vi "Create Dataset 2D Double.vi"(7 "Chunk size":i32, 8 "error in (no error)":errorcluster, 9 "Datatype":dbl[][](array[numeric]), 10 "Dataset name":string, 11 "Location id in":i32) -> (0 "error out":errorcluster, 3 "Dataset id":i32)   [LabVIEW 2014]
uses:
  Release/HDF5Tools.dll
  HDF5Tools.lvlib
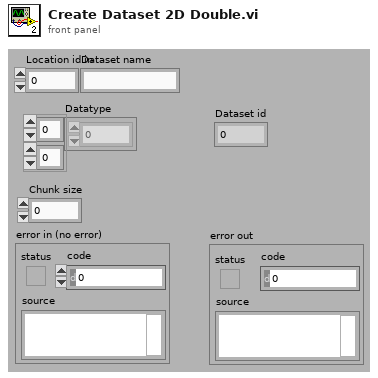
[diagram p1: front panel]
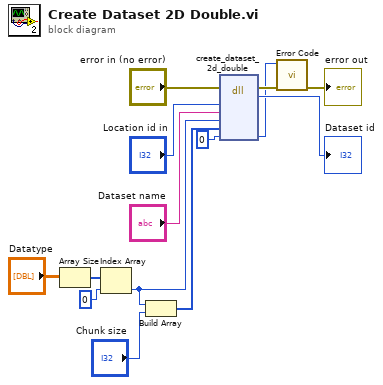
[diagram p0: block diagram]
diagram:
  n1 = Array Size(array="Datatype") -> (size(s)=w10:i32[])
  n2 = Index Array(array=w10, index=0) -> (element=w7:i32)
  n3 = Build Array(w7, "Chunk size") -> (w5:i32[])
  n4 = dll-call lib="C:/HDF5Tools/Release/HDF5Tools.dll" fn="create_dataset_2d_double"(error in="error in (no error)", "loc_id"="Location id in", "name"="Dataset name", "dim1"=w7, "chunks"=w5, "error"=0) -> (error out=w3:errorcluster, "dataset_id"=→"Dataset id":i32, "error"=w1:i32)  [unwired: 6 in, 1 out]
  n5 = call "Error Code.vi"("Error in"=w3, "Error code"=w1) -> ("Error out"=→"error out":errorcluster)  [unwired: 9 in]
